vi "KeyboardSimulation.vi"() -> ()   [LabVIEW 2016]
panel:
  in  "String Target":string
  in  "String":string
  in  "OK":bool
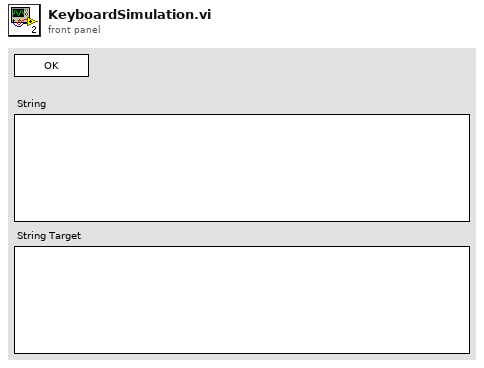
[diagram p1: front panel]
types:
  T1 = enum32{"Invalid", "Standard", "Closed", "Hidden", "Minimized", "Maximized"}
  T2 = enum32{"invalid app kind", "Development System", "Run Time System", "Student Edition", "Embedded LabVIEW", "Evaluation", "Custom"}
  T3 = cluster{"Core":cluster{"Current VI Reference":refnum<vi>, "Close Panel on Exit?":bool}, "Your Boolean data":bool, "Your string data":string}
  T4 = cluster{"Current VI Reference":refnum<vi>, "Close Panel on Exit?":bool}
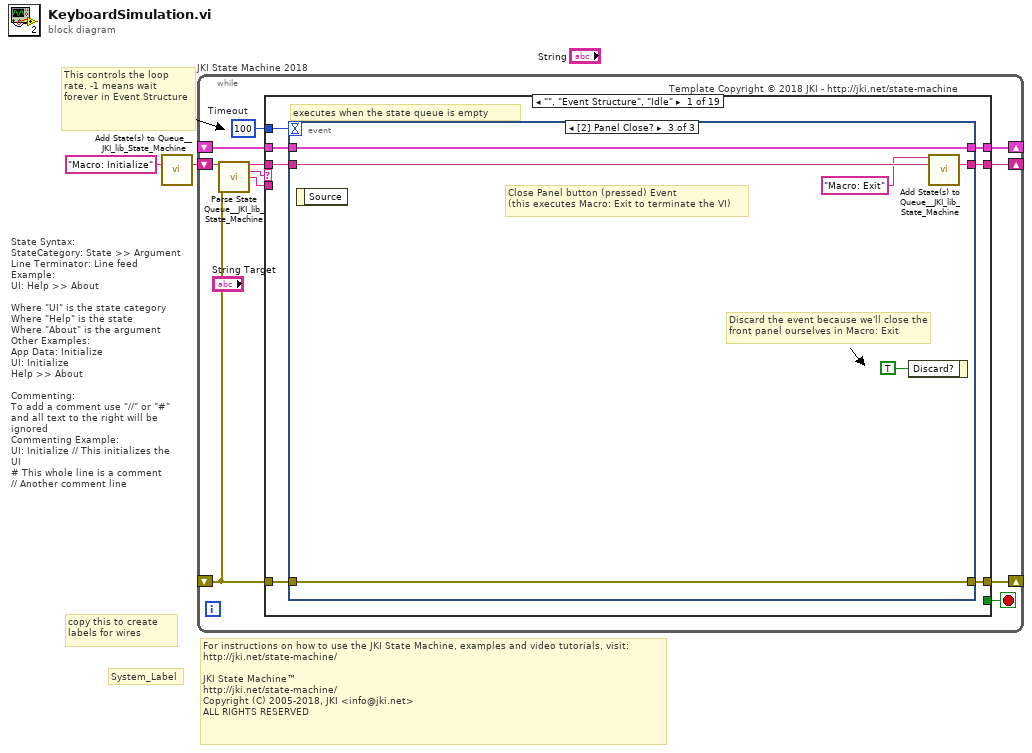
[diagram p0: block diagram]
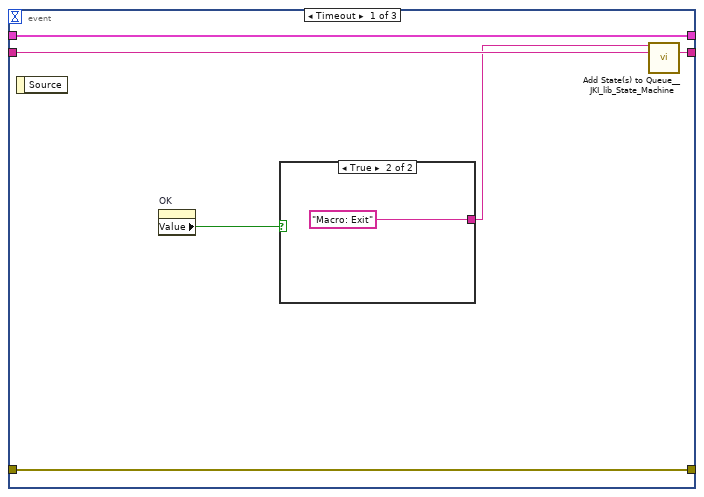
[diagram p2: hidden frame]
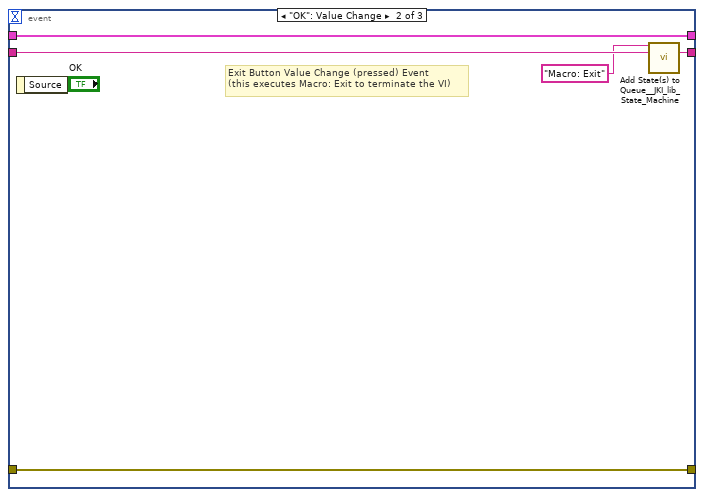
[diagram p4: hidden frame]
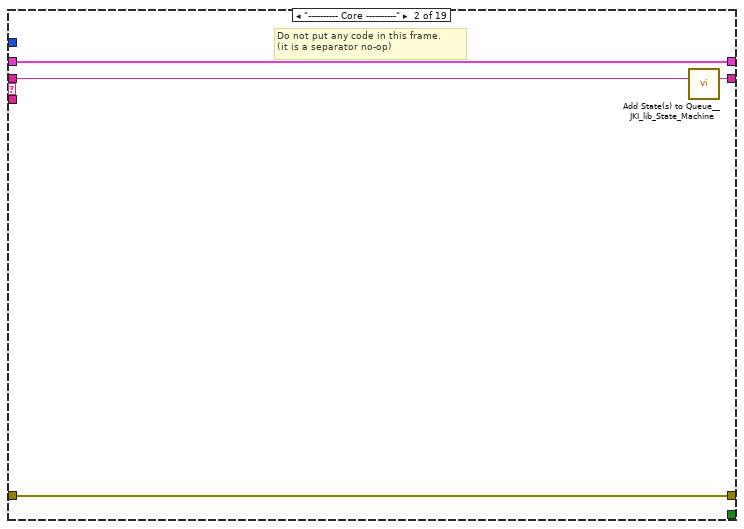
[diagram p5: hidden frame]
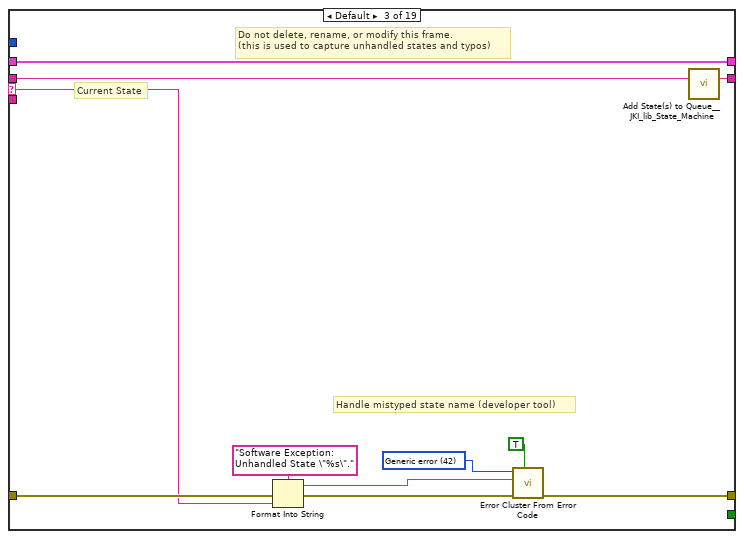
[diagram p6: hidden frame]
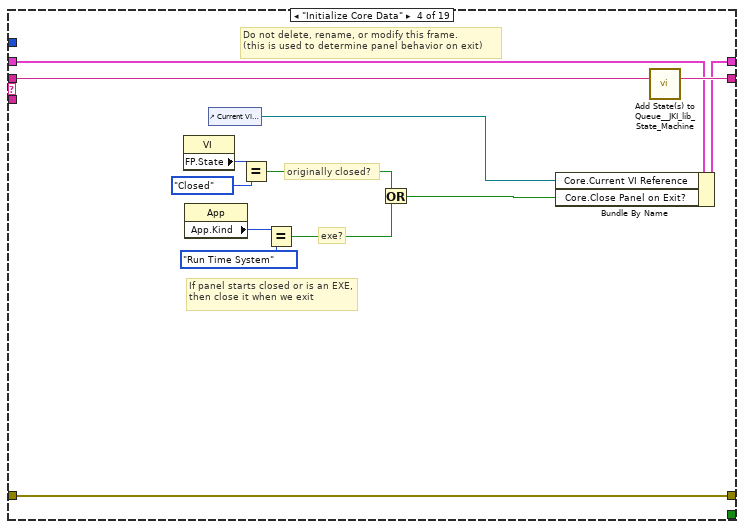
[diagram p7: hidden frame]
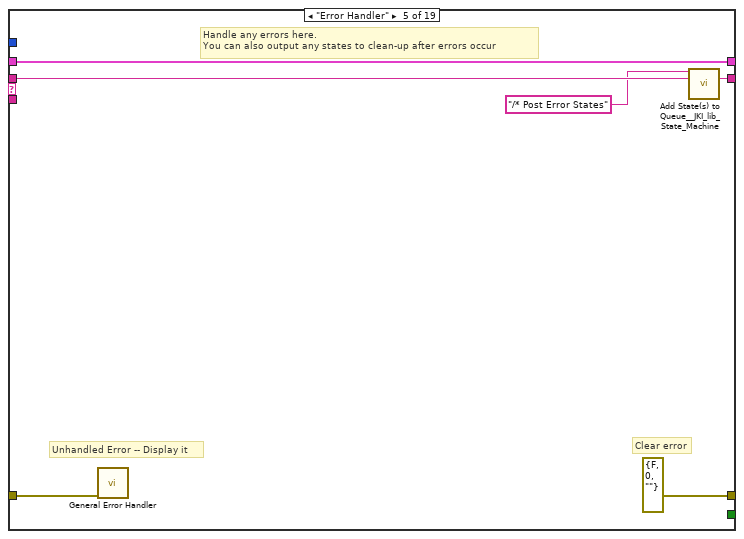
[diagram p8: hidden frame]
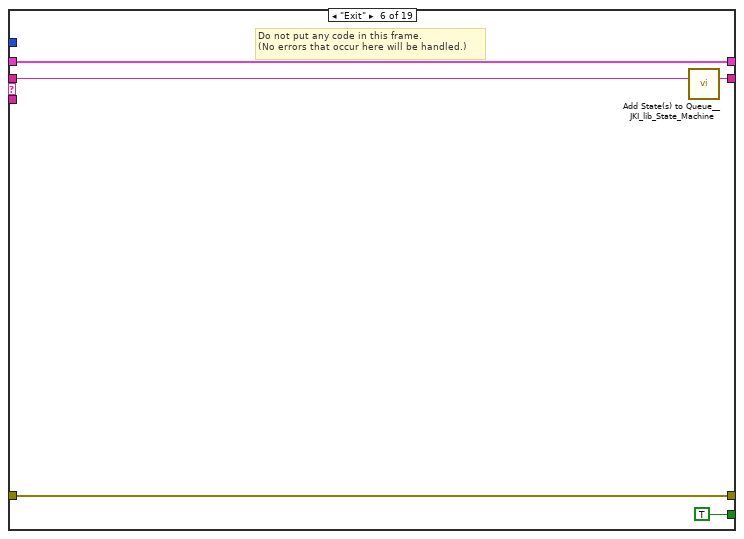
[diagram p9: hidden frame]
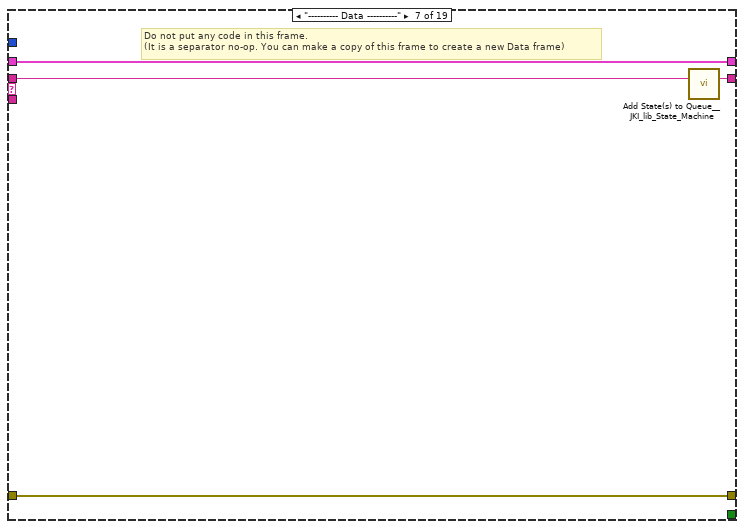
[diagram p10: hidden frame]
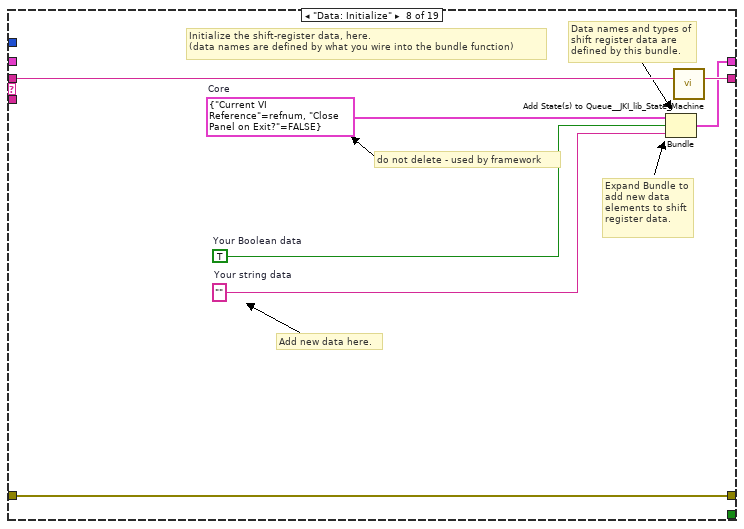
[diagram p11: hidden frame]
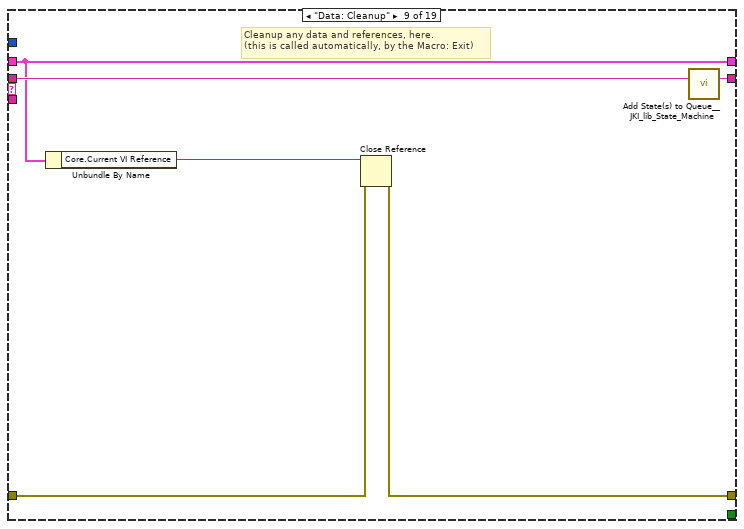
[diagram p12: hidden frame]
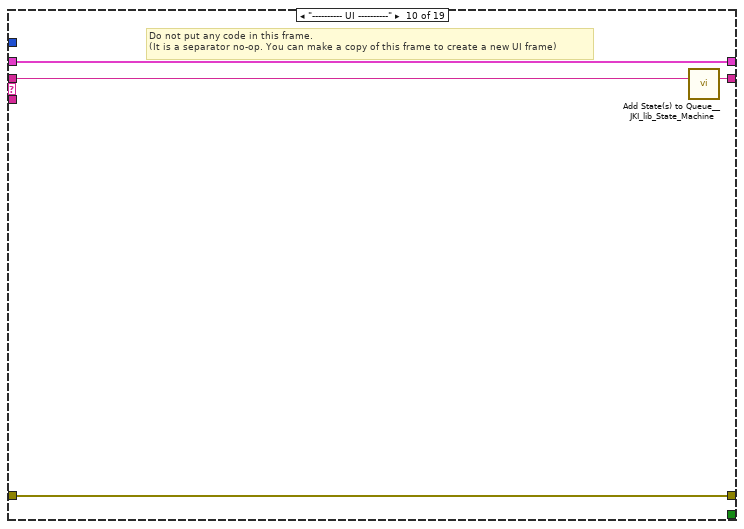
[diagram p13: hidden frame]
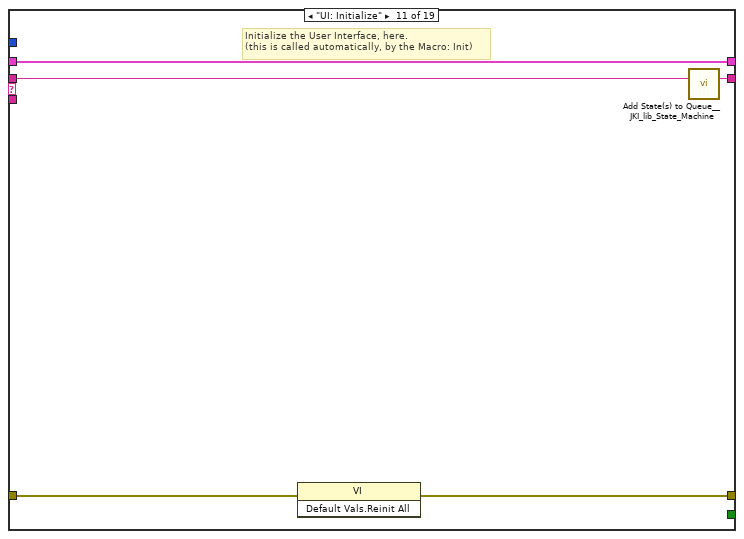
[diagram p14: hidden frame]
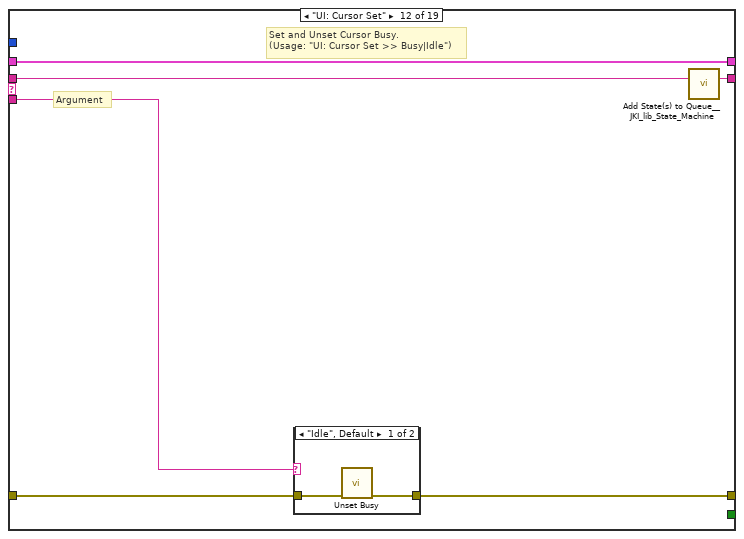
[diagram p15: hidden frame]
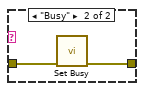
[diagram p16: hidden frame]
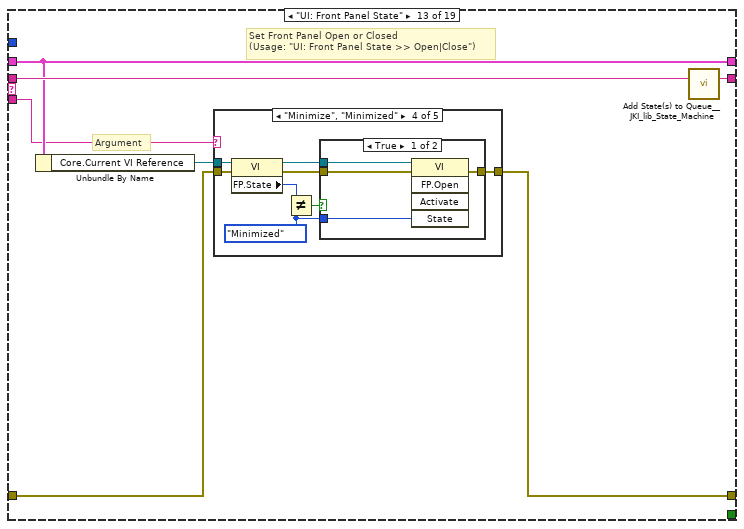
[diagram p17: hidden frame]
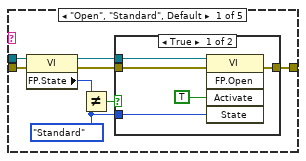
[diagram p18: hidden frame]
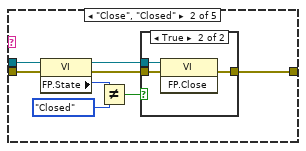
[diagram p20: hidden frame]
diagram:
  # "For instructions on how to use the JKI State Machine, examples and video tutorials, visit:\nhttp://jki.net/state-machine/\n\nJKI State Machine™\nhttp://jki.net/state-machine/\nCopyright (C) 2005-2018, JKI <info@jki.net>\nALL RIGHTS RESERVED"
  # "State Syntax:\nStateCategory: State >> Argument\nLine Terminator: Line feed\nExample:\nUI: Help >> About\n\nWhere \"UI\" is the state category\nWhere \"Help\" is the state\nWhere \"About\" is the argument\nOther Examples:\nApp Data: Initialize\nUI: Initialize\nHelp >> About\n\nCommenting:\nTo add a comment use \"//\" or \"#\" and all text to the right will be ignored\nCommenting Example:\nUI: Initialize // This initializes the UI\n# This whole line is a comment\n// Another comment line"
  # "copy this to create labels for wires"
  # "This controls the loop rate. -1 means wait forever in Event Structure"
  # "System_Label"
  n1 = call <vilib>:"Add State(s) to Queue__JKI_lib_State_Machine.vi"("State(s) in (\"\")"="Macro: Initialize") -> ("States Out"=w2:string)  [unwired: 14 in]
  n2 = while "JKI State Machine 2018" {
    shift-right: [w6] -> _
    shift-left: _ -> [w5]
    shift-right: [w9] -> _
    shift-left: _ -> [w3]
    shift-right: [w8] -> _
    shift-left: w2 -> [w10]
    stop <- w7 stop-if-true
    w4 = 100  # Timeout
    # "Template Copyright © 2018 JKI - http://jki.net/state-machine"
    n3 = call <vilib>:"Parse State Queue__JKI_lib_State_Machine.vi"("State Queue"=w10, "Error In (no error)"=w3) -> ("Remaining States"=w12:string, "Current State"=w13:string, "Arguments"=w11:string)  [unwired: 11 in]
    n4 = case shown="\"\", \"Event Structure\", \"Idle\"" w13 {
      selector: w13 -> [_ _ w43 _ _ _ _ _ _ _ _ _ _ _ _ _ _ _ _]
      tunnel: w12 -> [w20 w42 w47 w66 w72 w77 w81 w88 w94 w98 w103 w109 w120 w189 w194 w204 w208 w212 w216]
      tunnel: w11 -> [_ _ _ _ _ _ _ _ _ _ _ w104 w114 _ _ _ _ _ _]
      tunnel: w5 -> [w18 w39 w45 w59 w69 w75 w78 _ w89 w95 w101 w107 w116 w186 w191 w201 w205 w209 w213]
      tunnel: [w17 w40 w49 w63 errorcluster {"status"=FALSE, "code"=0, "source"=""} ("error out") w74 w79 w85 w90 w96 w99 w105 w117 w187 w192 w202 w206 w210 w214] -> w9
      tunnel: w3 -> [w16 w40 w48 w63 w68 w74 w79 w85 w91 w96 w100 w106 w118 w187 w192 w202 w206 w210 w214]
      tunnel: [w19 w41 w46 w65 w71 w76 w80 w87 w93 w97 w102 w108 w119 w188 w193 w203 w207 w211 w215] -> w8
      tunnel: [_ _ _ _ _ TRUE _ _ _ _ _ _ _ _ _ _ _ _ _] -> w7
      tunnel: [w15 w39 w45 w64 w69 w75 w78 w86 w89 w95 w101 w107 w116 w186 w191 w201 w205 w209 w213] -> w6
      tunnel: w4 -> [w14 _ _ _ _ _ _ _ _ _ _ _ _ _ _ _ _ _ _]
      frame "", "Event Structure", "Idle" {
        # "executes when the state queue is empty"
        n5 = event shown="[2] Panel Close?" {
          selector: _ -> [_ _ _]
          dyn-events: _ -> [_ _ _]
          timeout: w14 -> [_ _ _]
          tunnel: w20 -> [w26 w32 w38]
          tunnel: [w25 w31 w37] -> w19
          tunnel: w18 -> [w23 w29 w35]
          tunnel: [w24 w30 w36] -> w17
          tunnel: w16 -> [w24 w30 w36]
          tunnel: [w23 w29 w35] -> w15
          event Timeout {
            n6 = event-data() -> ()  [unwired: 1 in, 1 out]
            n7 = property on="OK" class="Bool (strict)"() -> ("Value"=w22:bool)  [unwired: 2 in, 2 out]
            n8 = case shown="True" w22 {
              tunnel: [_ "Macro: Exit"] -> w21
              frame False {
              }
              frame True {
              }
            }
            n9 = call <vilib>:"Add State(s) to Queue__JKI_lib_State_Machine.vi"("State(s) in Front (\"\")"=w21, "State(s) in (\"\")"=w26) -> ("States Out"=w25:string)  [unwired: 13 in]
          }
          event "OK": Value Change {
            # "Exit Button Value Change (pressed) Event\n(this executes Macro: Exit to terminate the VI)"
            n10 = event-data() -> ()  [unwired: 1 in, 1 out]
            n11 = call <vilib>:"Add State(s) to Queue__JKI_lib_State_Machine.vi"("State(s) in Front (\"\")"="Macro: Exit", "State(s) in (\"\")"=w32) -> ("States Out"=w31:string)  [unwired: 13 in]
          }
          event Panel Close? {
            # "Discard the event because we'll close the front panel ourselves in Macro: Exit"
            # "Close Panel button (pressed) Event\n(this executes Macro: Exit to terminate the VI)"
            n12 = event-data() -> ()  [unwired: 1 in, 1 out]
            n13 = event-data("Discard?"=TRUE) -> ()  [unwired: 1 in, 1 out]
            n14 = call <vilib>:"Add State(s) to Queue__JKI_lib_State_Machine.vi"("State(s) in Front (\"\")"="Macro: Exit", "State(s) in (\"\")"=w38) -> ("States Out"=w37:string)  [unwired: 13 in]
          }
        }
      }
      frame "---------- Core ----------" {
        # "Do not put any code in this frame.\n(it is a separator no-op)"
        n15 = call <vilib>:"Add State(s) to Queue__JKI_lib_State_Machine.vi"("State(s) in (\"\")"=w42) -> ("States Out"=w41:string)  [unwired: 14 in]
      }
      frame Default {
        w52 = 42 items=["No error", "Argument error", "Memory is full", "Out of zone", "End of file", "File already open", "Generic file I/O error", "File not found", "File permission error", "Disk is full", "Duplicate path", "Too many files open", "System feature not enabled", "Resource file not found", "Cannot add resource", "Resource not found", "Image not found", "Image memory error", "Pen does not exist", "Config type invalid", "Config token not found", "Config parse error", "Config memory error", "Bad external code format", "Bad external code offset", "External code not present", "Null window", "Destroy window error", "Null menu", "Print aborted", "Bad print record", "Print driver error", "Windows error during printing", "Memory error during printing", "Print dialog error", "Generic print error", "Invalid device refnum", "Device not found", "Device parameter error", "Device unit error", "Cannot open device", "Device call aborted", "Generic error", "Cancelled by user", "Object ID too low", "Object ID too high", "Object not in heap", "Unknown heap", "Unknown object (invalid DefProc)", "Unknown object (DefProc not in table)", "Message out of range", "Invalid (null) method", "Unknown message", "Manager call not supported", "Bad address", "Network operation in progress", "Network operation timed out", "Connection is busy", "Network attribute not supported", "Network error", "Address in use", "System out of memory", "Connection aborted", "Connection refused", "Not connected", "Already connected", "Connection closed", "Initialization error (interapplication manager)", "Bad occurrence", "Wait on unbound occurrence handler", "Occurrence queue overflow", "Datalog type conflict", "Unused", "Unrecognized type (interapplication manager)", "Memory corrupt", "Failed to make temporary DLL", "Old CIN version", "Drag socket not found", "Failed to load drop-object", "Failed to register OLE object", "Failed to release OLE object", "Format specifier type mismatch", "Unknown format specifier", "Too few format specifiers", "Too many format specifiers", "Scan failed", "Newer CIN version", "Error converting to variant", "Runtime menu error", "Password tampered", "Variant attribute not found", "Incompatible variant data type", "Event data is not available", "Event Store is not present", "Occurrence is not found", "Event Queue is not created", "Event info is not available", "Refnum passed is NULL", "Error retrieving Class GUID", "Error retrieving CoClass GUID", "Error retrieving TypeLib GUID.", "Bad built application magic bytes.", "Specific driver is different from the specific driver associated with the Logical Name.", "There is no session opened to the class driver.", "Max Error", "MAX - Error with config objects", "MAX - Error loading configuration", "MAX - Group not supported"]
        # "Current State"
        # "Do not delete, rename, or modify this frame.\n(this is used to capture unhandled states and typos)"
        # "Handle mistyped state name (developer tool)"
        n16 = Format Into String(format string="Software Exception: Unhandled State \"%s\"." ("message"), error in=w48, w43) -> (resulting string=w51:string, error out=w50:errorcluster)  [unwired: 1 in]
        n17 = call <vilib>:"Error Cluster From Error Code.vi"("show call chain? (False)"=TRUE, "error in (no error)"=w50, "error message (\"\")"=w51, "error code (0)"=w52) -> ("error out"=w49:errorcluster)  [unwired: 5 in]
        n18 = call <vilib>:"Add State(s) to Queue__JKI_lib_State_Machine.vi"("State(s) in (\"\")"=w47) -> ("States Out"=w46:string)  [unwired: 14 in]
      }
      frame "Initialize Core Data" {
        # "Do not delete, rename, or modify this frame.\n(this is used to determine panel behavior on exit)"
        # "originally closed?"
        # "exe?"
        # "If panel starts closed or is an EXE, then close it when we exit"
        n19 = property class="VI"() -> ("FP.State"=w56:T1)  [unwired: 2 in, 2 out]
        n20 = property class="App"() -> ("App.Kind"=w62:T2)  [unwired: 2 in, 2 out]
        n21 = control-ref of="Current VI Reference"() -> (w57:refnum<vi>)
        n22 = Equal?(x=w56, y=T1."Closed" ("Front Panel Window:State")) -> (x = y?=w54:bool)
        n23 = Equal?(x=w62, y=T2."Run Time System" ("Application:Kind")) -> (x = y?=w60:bool)
        n24 = Or(x=w54, y=w60) -> (x .or. y?=w58:bool)
        n25 = Bundle By Name(cluster=w59, "Core.Current VI Reference"=w57, "Core.Close Panel on Exit?"=w58) -> (w64:T3)
        n26 = call <vilib>:"Add State(s) to Queue__JKI_lib_State_Machine.vi"("State(s) in (\"\")"=w66) -> ("States Out"=w65:string)  [unwired: 14 in]
      }
      frame "Error Handler" {
        # "Unhandled Error -- Display it"
        # "Handle any errors here.\nYou can also output any states to clean-up after errors occur"
        # "Clear error"
        n27 = call <vilib>:"General Error Handler.vi"("error in (no error)"=w68) -> ()  [unwired: 10 in, 5 out]
        n28 = call <vilib>:"Add State(s) to Queue__JKI_lib_State_Machine.vi"("State(s) in Front (\"\")"="/* Post Error States", "State(s) in (\"\")"=w72) -> ("States Out"=w71:string)  [unwired: 13 in]
      }
      frame "Exit" {
        # "Do not put any code in this frame.\n(No errors that occur here will be handled.)"
        n29 = call <vilib>:"Add State(s) to Queue__JKI_lib_State_Machine.vi"("State(s) in (\"\")"=w77) -> ("States Out"=w76:string)  [unwired: 14 in]
      }
      frame "---------- Data ----------" {
        # "Do not put any code in this frame.\n(It is a separator no-op. You can make a copy of this frame to create a new Data frame)"
        n30 = call <vilib>:"Add State(s) to Queue__JKI_lib_State_Machine.vi"("State(s) in (\"\")"=w81) -> ("States Out"=w80:string)  [unwired: 14 in]
      }
      frame "Data: Initialize" {
        w82 = T4 {"Current VI Reference"=refnum, "Close Panel on Exit?"=FALSE}  # Core
        w84 = TRUE  # Your Boolean data
        w83 = ""  # Your string data
        # "do not delete - used by framework"
        # "Expand Bundle to add new data elements to shift register data."
        # "Add new data here."
        # "Data names and types of shift register data are defined by this bundle."
        # "Initialize the shift-register data, here.\n(data names are defined by what you wire into the bundle function)"
        n31 = Bundle("Core"=w82, "Your Boolean data"=w84, "Your string data"=w83) -> (w86:T3)  [unwired: 1 in]
        n32 = call <vilib>:"Add State(s) to Queue__JKI_lib_State_Machine.vi"("State(s) in (\"\")"=w88) -> ("States Out"=w87:string)  [unwired: 14 in]
      }
      frame "Data: Cleanup" {
        # "Cleanup any data and references, here.\n(this is called automatically, by the Macro: Exit)"
        n33 = Unbundle By Name(w89) -> ("Core.Current VI Reference"=w92:refnum<vi>)
        n34 = Close Reference(reference=w92, error in (no error)=w91) -> (error out=w90:errorcluster)
        n35 = call <vilib>:"Add State(s) to Queue__JKI_lib_State_Machine.vi"("State(s) in (\"\")"=w94) -> ("States Out"=w93:string)  [unwired: 14 in]
      }
      frame "---------- UI ----------" {
        # "Do not put any code in this frame.\n(It is a separator no-op. You can make a copy of this frame to create a new UI frame)"
        n36 = call <vilib>:"Add State(s) to Queue__JKI_lib_State_Machine.vi"("State(s) in (\"\")"=w98) -> ("States Out"=w97:string)  [unwired: 14 in]
      }
      frame "UI: Initialize" {
        # "Initialize the User Interface, here.\n(this is called automatically, by the Macro: Init)"
        n37 = invoke class="VI" method="Default Vals.Reinit All"(error in=w100) -> (error out=w99:errorcluster)  [unwired: 2 in, 2 out]
        n38 = call <vilib>:"Add State(s) to Queue__JKI_lib_State_Machine.vi"("State(s) in (\"\")"=w103) -> ("States Out"=w102:string)  [unwired: 14 in]
      }
      frame "UI: Cursor Set" {
        # "Argument"
        # "Set and Unset Cursor Busy.\n(Usage: \"UI: Cursor Set >> Busy|Idle\")"
        n39 = case shown="\"Idle\", Default" w104 {
          tunnel: w106 -> [w111 w113]
          tunnel: [w110 w112] -> w105
          frame "Idle", Default {
            n40 = call <vilib>:"Unset Busy.vi"("error in (no error)"=w111) -> ("error out"=w110:errorcluster)  [unwired: 10 in]
          }
          frame "Busy" {
            n41 = call <vilib>:"Set Busy.vi"("error in (no error)"=w113) -> ("error out"=w112:errorcluster)  [unwired: 9 in, 1 out]
          }
        }
        n42 = call <vilib>:"Add State(s) to Queue__JKI_lib_State_Machine.vi"("State(s) in (\"\")"=w109) -> ("States Out"=w108:string)  [unwired: 14 in]
      }
      frame "UI: Front Panel State" {
        # "Argument"
        # "Set Front Panel Open or Closed\n(Usage: \"UI: Front Panel State >> Open|Close\")"
        n43 = Unbundle By Name(w116) -> ("Core.Current VI Reference"=w115:refnum<vi>)
        n44 = case shown="\"Minimize\", \"Minimized\"" w114 {
          tunnel: w118 -> [w126 w141 w152 w165 w178]
          tunnel: [w128 w142 w154 w167 w180] -> w117
          tunnel: w115 -> [w127 w139 w153 w166 w179]
          frame "Open", "Standard", Default {
            w121 = T1."Standard" ("State")
            n45 = property class="VI"(reference=w127, error in=w126) -> (reference out=w124:refnum<vi>, error out=w125:errorcluster, "FP.State"=w123:T1)
            n46 = Not Equal?(x=w123, y=w121) -> (x != y?=w122:bool)
            n47 = case shown="True" w122 {
              tunnel: [w132 w134] -> w128
              tunnel: w125 -> [w131 w134]
              tunnel: w124 -> [w130 _]
              tunnel: w121 -> [w129 _]
              frame True {
                n48 = invoke class="VI" method="FP.Open"(reference=w130, error in=w131, "Activate"=TRUE, "State"=w129) -> (error out=w132:errorcluster)  [unwired: 1 in, 4 out]
              }
              frame False {
              }
            }
          }
          frame "Close", "Closed" {
            n49 = property class="VI"(reference=w139, error in=w141) -> (reference out=w138:refnum<vi>, error out=w140:errorcluster, "FP.State"=w136:T1)
            n50 = Not Equal?(x=w136, y=T1."Closed" ("Front Panel Window:State")) -> (x != y?=w135:bool)
            n51 = case shown="True" w135 {
              tunnel: [w143 w146] -> w142
              tunnel: w140 -> [w143 w145]
              tunnel: w138 -> [_ w144]
              frame False {
              }
              frame True {
                n52 = invoke class="VI" method="FP.Close"(reference=w144, error in=w145) -> (error out=w146:errorcluster)  [unwired: 1 in, 2 out]
              }
            }
          }
          frame "Hidden", "Hide" {
            w147 = T1."Hidden" ("State")
            n53 = property class="VI"(reference=w153, error in=w152) -> (reference out=w150:refnum<vi>, error out=w151:errorcluster, "FP.State"=w149:T1)
            n54 = Not Equal?(x=w149, y=w147) -> (x != y?=w148:bool)
            n55 = case shown="True" w148 {
              tunnel: [w158 w159] -> w154
              tunnel: w151 -> [w157 w159]
              tunnel: w150 -> [w156 _]
              tunnel: w147 -> [w155 _]
              frame True {
                n56 = invoke class="VI" method="FP.Open"(reference=w156, error in=w157, "State"=w155) -> (error out=w158:errorcluster)  [unwired: 2 in, 4 out]
              }
              frame False {
              }
            }
          }
          frame "Minimize", "Minimized" {
            w160 = T1."Minimized" ("State")
            n57 = property class="VI"(reference=w166, error in=w165) -> (reference out=w163:refnum<vi>, error out=w164:errorcluster, "FP.State"=w162:T1)
            n58 = Not Equal?(x=w162, y=w160) -> (x != y?=w161:bool)
            n59 = case shown="True" w161 {
              tunnel: [w171 w172] -> w167
              tunnel: w164 -> [w170 w172]
              tunnel: w163 -> [w169 _]
              tunnel: w160 -> [w168 _]
              frame True {
                n60 = invoke class="VI" method="FP.Open"(reference=w169, error in=w170, "State"=w168) -> (error out=w171:errorcluster)  [unwired: 2 in, 4 out]
              }
              frame False {
              }
            }
          }
          frame "Maximize", "Maximized" {
            w173 = T1."Maximized" ("State")
            n61 = property class="VI"(reference=w179, error in=w178) -> (reference out=w176:refnum<vi>, error out=w177:errorcluster, "FP.State"=w175:T1)
            n62 = Not Equal?(x=w175, y=w173) -> (x != y?=w174:bool)
            n63 = case shown="True" w174 {
              tunnel: [w184 w185] -> w180
              tunnel: w177 -> [w183 w185]
              tunnel: w176 -> [w182 _]
              tunnel: w173 -> [w181 _]
              frame True {
                n64 = invoke class="VI" method="FP.Open"(reference=w182, error in=w183, "State"=w181) -> (error out=w184:errorcluster)  [unwired: 2 in, 4 out]
              }
              frame False {
              }
            }
          }
        }
        n65 = call <vilib>:"Add State(s) to Queue__JKI_lib_State_Machine.vi"("State(s) in (\"\")"=w120) -> ("States Out"=w119:string)  [unwired: 14 in]
      }
      frame "---------- Macro ----------" {
        # "Do not put any code in this frame.\n(It is a separator no-op. You can make a copy of this frame to create a new Macro frame)"
        n66 = call <vilib>:"Add State(s) to Queue__JKI_lib_State_Machine.vi"("State(s) in (\"\")"=w189) -> ("States Out"=w188:string)  [unwired: 14 in]
      }
      frame "Macro: Initialize" {
        w190 = "Data: Initialize\nInitialize Core Data\nUI: Initialize\nUI: Front Panel State >> Open"  # Data: Initialize Initialize Core Data UI: Initialize UI: Front Panel State >> Open
        # "Initialization Macro\n(This is called once, when the VI starts)"
        n67 = call <vilib>:"Add State(s) to Queue__JKI_lib_State_Machine.vi"("State(s) in Front (\"\")"=w190, "State(s) in (\"\")"=w194) -> ("States Out"=w193:string)  [unwired: 13 in]
      }
      frame "Macro: Exit" {
        # "Exit Macro\n(This is called once, when the VI exits)"
        n68 = Unbundle By Name(w201) -> ("Core.Close Panel on Exit?"=w200:bool)
        n69 = Select(t="UI: Front Panel State >> Close", s=w200, f="") -> (s? t:f=w197:string)
        n70 = call <vilib>:"Add State(s) to Queue__JKI_lib_State_Machine.vi"("State(s) in (\"\")"=w197, "State(s) at Back (\"\")"="Data: Cleanup\nExit") -> ("States Out"=w195:string)  [unwired: 13 in]
        n71 = call <vilib>:"Add State(s) to Queue__JKI_lib_State_Machine.vi"("State(s) in Front (\"\")"=w195, "State(s) in (\"\")"=w204) -> ("States Out"=w203:string)  [unwired: 13 in]
      }
      frame "---------- New Category ----------" {
        # "Template Separator\n(You can make a copy of, or modify, this frame)"
        n72 = call <vilib>:"Add State(s) to Queue__JKI_lib_State_Machine.vi"("State(s) in (\"\")"=w208) -> ("States Out"=w207:string)  [unwired: 14 in]
      }
      frame "New Category: 1" {
        # "Your code here.\n(You can make a copy of, or modify, this frame)"
        n73 = call <vilib>:"Add State(s) to Queue__JKI_lib_State_Machine.vi"("State(s) in (\"\")"=w212) -> ("States Out"=w211:string)  [unwired: 14 in]
      }
      frame "New Category: 2" {
        # "Your code here.\n(You can make a copy of, or modify, this frame)"
        n74 = call <vilib>:"Add State(s) to Queue__JKI_lib_State_Machine.vi"("State(s) in (\"\")"=w216) -> ("States Out"=w215:string)  [unwired: 14 in]
      }
    }
  }
